vi "tiffOpenForRead.vi"(8 "error in (no error)":errorcluster, 11 "Path":path) -> (0 "error out":errorcluster, 3 "TiffOut":refnum<k24>)   [LabVIEW 2022 SP3]
doc: "Opens file for writing tiffs."
uses:
  C:/Nuget/BitMiracle.LibTiff.NET.2.4.649/lib/net40/BitMiracle.LibTiff.NET.dll
  Nuget/BitMiracle.LibTiff.NET.2.4.649/lib/net40/BitMiracle.LibTiff.NET.dll
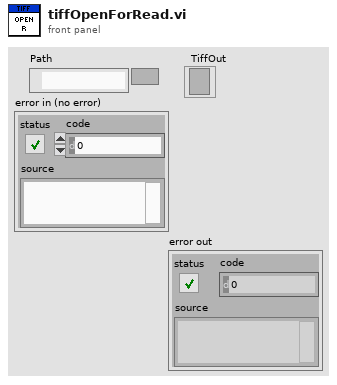
[diagram p1: front panel]
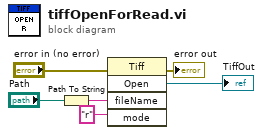
[diagram p0: block diagram]
diagram:
  n1 = Path To String(path="Path") -> (string=w6:string)
  n2 = invoke class="Tiff" method="Open"(error in="error in (no error)", "fileName"=w6, "mode"="r") -> (error out=→"error out":errorcluster, "Open"=→"TiffOut":refnum<k24>)  [unwired: 2 in, 3 out]
